vi "Global_HW Status.vi"() -> ()   [LabVIEW 2017, in "Shooter.lvlib"]
uses:
  Shooter.lvlib
  TypeDefs/Cluster_SRX Status With Encoder.ctl
  TypeDefs/Cluster_SRX Limit Switches.ctl
panel:
  out "HW_Hood Limits":T1
  out "HW_Hood Status":T2
  out "HW_Wheel Status":T2
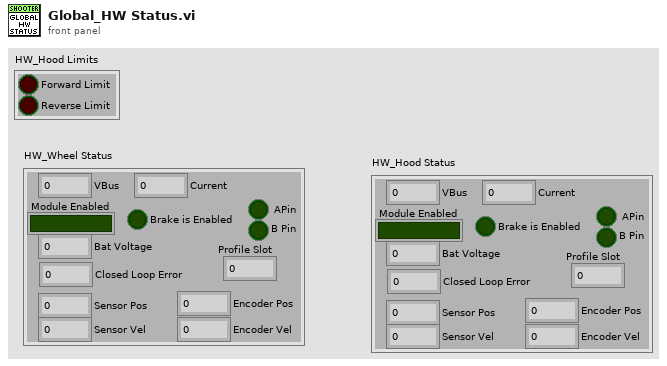
[diagram p1: front panel]
types:
  T1 = typedef "Cluster_SRX Limit Switches.ctl" = cluster{"Forward Limit":bool, "Reverse Limit":bool}
  T2 = typedef "Cluster_SRX Status With Encoder.ctl" = cluster{"VBus ":dbl, "Module Enabled":bool, "Closed Loop Error":dbl, "Sensor Pos":dbl, "Sensor Vel":dbl, "Current":dbl, "Brake is Enabled":bool, "Encoder Pos":dbl, "Encoder Vel":dbl, " APin":bool, "B Pin":bool, "Bat Voltage":dbl, "Profile Slot":dbl}
diagram:
